vi "DisconnectAll.vi"(0 "reference in":refnum<class "Switch_Keysight_34934A.lvclass">, 5 "error in (no error)":errorcluster) -> (14 "reference in":refnum<class "Switch_Keysight_34934A.lvclass">, 19 "error out":errorcluster)   [LabVIEW 2022 SP3, in "Switch_Keysight_34934A.lvlib" / "Switch_Keysight_34934A.lvclass"]
uses:
  Switch_Keysight_34934A.lvclass
  Matrix.ctl
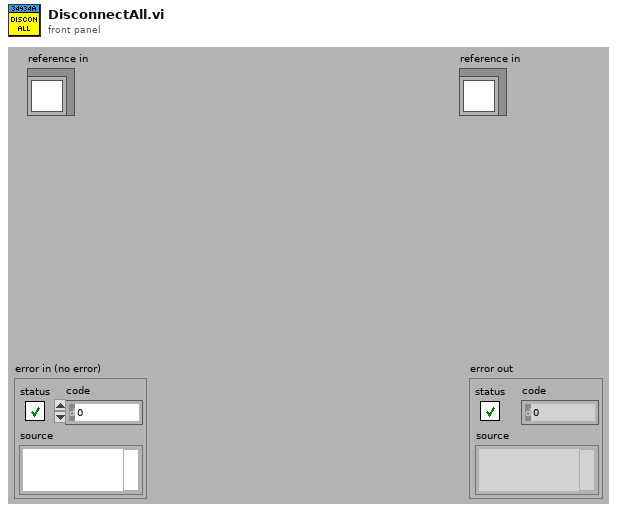
[diagram p1: front panel]
types:
  T1 = typedef "Switch_Keysight_34934A.lvlib/Switch_Keysight_34934A.lvclass/Matrix.ctl" = enum16{"M1H", "M2H", "M1L", "M2L"}
  T2 = typedef "Switch_Keysight_34934A.lvlib/Switch_Keysight_34934A.lvclass/ObjectAttributes.ctl" = cluster{"Config":T3, "VISA ref":refnum<visa-resource-name>, "M1H":bool[][], "M2H":bool[][], "M1L":bool[][], "M2L":bool[][], "route":string, "State":bool[], "StateModBit":bool[], "UpdateEvent":refnum<user-event>}
  T3 = typedef "Switch_Keysight_34934A.lvlib/Switch_Keysight_34934A.lvclass/Config.ctl" = cluster{"VISA":refnum<visa-resource-name>, "Slot":i32, "SwitchMap":cluster{"Name":string, "Route":string[], "UnRoute":string[], "Description":string, "Group":string, "IsGroup":bool}[], "Sim":bool}
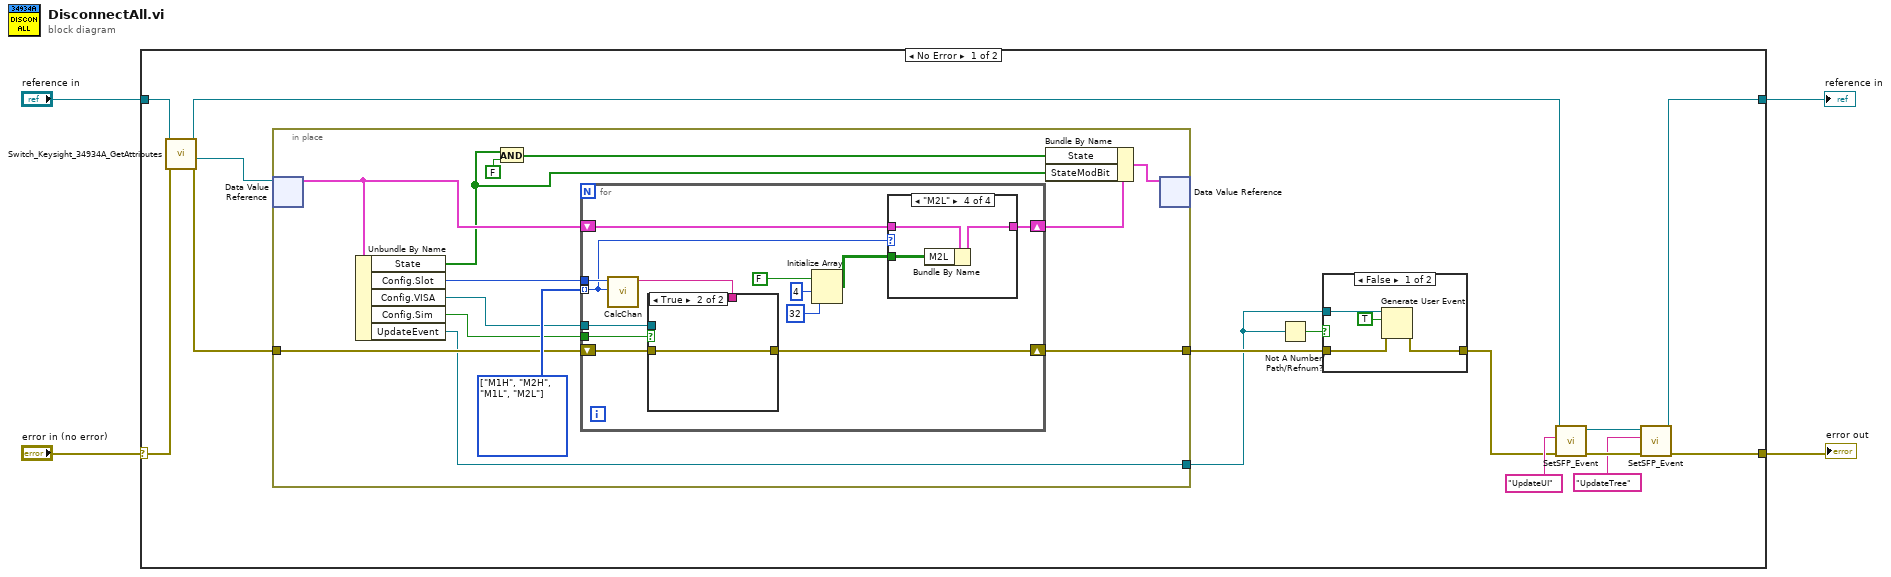
[diagram p0: block diagram]
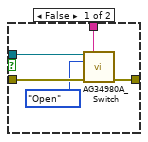
[diagram p3: hidden frame]
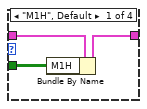
[diagram p4: hidden frame]
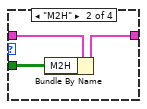
[diagram p5: hidden frame]
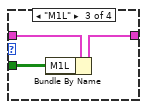
[diagram p6: hidden frame]
diagram:
  n1 = case shown="No Error" "error in (no error)" {
    selector: "error in (no error)" -> [w17 w70]
    tunnel: [w12 w70] -> w3
    tunnel: [w10 w69] -> w1
    tunnel: "reference in" -> [w16 w69]
    frame No Error {
      n2 = call "Switch_Keysight_34934A_GetAttributes.vi"("error in (no error)"=w17, "reference in"=w16) -> ("error out"=w15:errorcluster, "DataRef"=w14:refnum<data-value>, "reference out"=w18:refnum<class "Switch_Keysight_34934A.lvclass">)  [unwired: 6 in, 1 out]
      n3 = in-place {
        in-place-border: w15 -> [w33]
        in-place-border: [w37] -> w7
        in-place-border: [w25] -> w5
        w35 = T1[] [enum."M1H", enum."M2H", enum."M1L", enum."M2L"] items=["M1H", "M2H", "M1L", "M2L"]
        n4 = in-place-dvr #1(w14) -> (w34:T2)  [unwired: 1 out]
        n5 = Unbundle By Name(w34) -> ("State"=w26:bool[], "Config.Slot"=w36:i32, "Config.VISA"=w32:refnum<visa-resource-name>, "Config.Sim"=w31:bool, "UpdateEvent"=w25:refnum<user-event>)
        n6 = And(x=w26, y=FALSE) -> (x .and. y?=w27:bool[])
        n7 = for {
          tunnel: w36 -> [w49]
          shift-right: [w43] -> w37
          shift-left: w33 -> [w50]
          tunnel: w35 -> [w47] mode=indexing
          shift-right: [w45] -> w29
          shift-left: w34 -> [w46]
          tunnel: w32 -> [w44]
          tunnel: w31 -> [w38]
          n8 = call "CalcChan.vi"("Matrix"=w47, "Slot"=w49) -> ("Matrix Chans"=w48:string)  [unwired: 8 in, 1 out]
          n9 = case shown="True" w38 {
            tunnel: w50 -> [w55 w56]
            tunnel: w48 -> [w53 _]
            tunnel: w44 -> [w52 _]
            tunnel: [w51 w56] -> w43
            frame False {
              n10 = call "AG34980A_Switch.vi"("VISA resource name"=w52, "Channel List"=w53, "Open/Close (0:Close)"=enum16{"Close", "Open"}."Open", "error in (no error)"=w55) -> ("error out"=w51:errorcluster)  [unwired: 9 in, 2 out]
            }
            frame True {
            }
          }
          n11 = Initialize Array(FALSE, 4 ("dimension size"), 32 ("dimension size")) -> (w39:bool[][])
          n12 = case shown="\"M2L\"" w47 {
            tunnel: w46 -> [w59 w62 w65 w68]
            tunnel: [w58 w61 w64 w67] -> w45
            tunnel: w39 -> [w57 w60 w63 w66]
            frame "M1H", Default {
              n13 = Bundle By Name(cluster=w59, "M1H"=w57) -> (w58:T2)
            }
            frame "M2H" {
              n14 = Bundle By Name(cluster=w62, "M2H"=w60) -> (w61:T2)
            }
            frame "M1L" {
              n15 = Bundle By Name(cluster=w65, "M1L"=w63) -> (w64:T2)
            }
            frame "M2L" {
              n16 = Bundle By Name(cluster=w68, "M2L"=w66) -> (w67:T2)
            }
          }
        }
        n17 = Bundle By Name(cluster=w29, "State"=w27, "StateModBit"=w26) -> (w28:T2)
        n18 = in-place-dvr #1(w28) -> ()  [unwired: 2 out]
      }
      n19 = Not A Number/Path/Refnum?(number/path/refnum=w5) -> (NaN/Path/Refnum?=w8:bool)
      n20 = case shown="False" w8 {
        tunnel: w7 -> [w21 w24]
        tunnel: [w22 w24] -> w6
        tunnel: w5 -> [w23 _]
        frame False {
          n21 = Generate User Event(user event=w23, event data cluster=TRUE ("event data"), error in=w21) -> (error out=w22:errorcluster)  [unwired: 1 in, 1 out]
        }
        frame True {
        }
      }
      n22 = call-dynamic "SetSFP_Event.vi"("error in (no error)"=w6, "msg"="UpdateUI", "reference in"=w18) -> ("error out"=w13:errorcluster, "reference out"=w11:refnum<class "Switch_Keysight_34934A.lvclass">)  [unwired: 7 in]
      n23 = call-dynamic "SetSFP_Event.vi"("error in (no error)"=w13, "msg"="UpdateTree", "reference in"=w11) -> ("error out"=w12:errorcluster, "reference out"=w10:refnum<class "Switch_Keysight_34934A.lvclass">)  [unwired: 7 in]
    }
    frame Error {
    }
  }
  "error out" <- w3
  "reference in" <- w1
